vi "picoRunBlock.vi"(8 "error in (no error)":errorcluster, 9 "timebase":u32, 10 "postTriggerSamples":u32, 11 "Handle In":i16) -> (0 "error out":errorcluster, 2 "postTriggerSamples Out":u32, 3 "handle":i16)   [LabVIEW 2011]
uses:
  PS2000a.dll
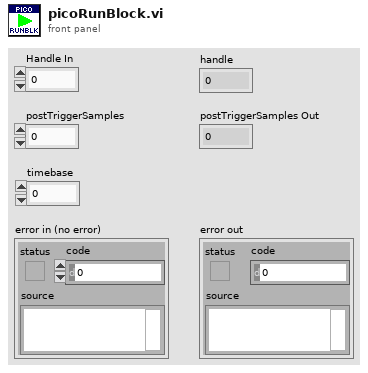
[diagram p1: front panel]
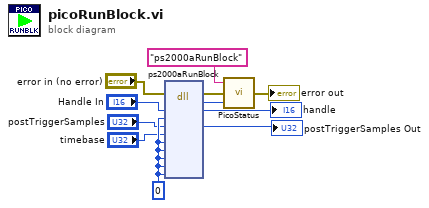
[diagram p0: block diagram]
diagram:
  w11 = 0 ("pParameter")
  n1 = dll-call lib="ps2000a.dll" fn="ps2000aRunBlock" ("ps3000.dll:_ps3000_open_unit@0")(error in="error in (no error)", "handle"="Handle In", "preTriggerSamples"=w11, "postTriggerSamples"="postTriggerSamples", "timebase"="timebase", "oversample"=w11, "timeindisposed"=w11, "segmentIndex"=w11, "lpReady"=w11, "pParameter"=w11) -> (error out=w3:errorcluster, "PICO_STATUS"=w2:i32, "handle"=→"handle":i16, "postTriggerSamples"=→"postTriggerSamples Out":u32)  [unwired: 9 in, 1 out]
  n2 = call "PicoStatus.vi"("PICO STATUS"=w2, "error in"=w3, "source"="ps2000aRunBlock") -> ("error out"=→"error out":errorcluster)
